vi "read full file.vi"(8 "error in":errorcluster, 11 "file path":path) -> (0 "error out":errorcluster, 2 "data":string)   [LabVIEW 2013, in "NISE Tools File IO.lvlib"]
doc: "Reads the full binary contents of a file."
uses:
  NISE Tools File IO.lvlib
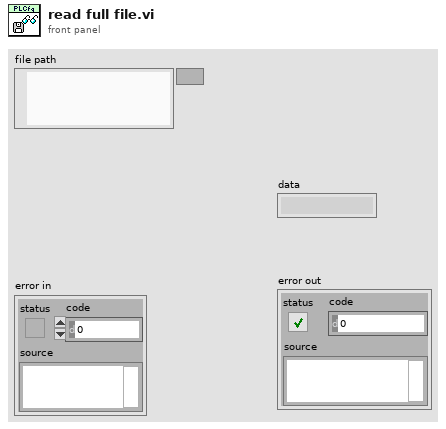
[diagram p1: front panel]
types:
  T1 = enum16{"open", "replace", "create", "open or create", "replace or create", "replace or create with confirmation"}
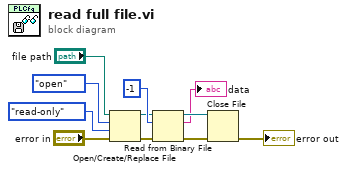
[diagram p0: block diagram]
diagram:
  n1 = Open/Create/Replace File(file path (use dialog)="file path", error in="error in", operation (0:open)=T1."open", access (0:read/write)=enum16{"read/write", "read-only", "write-only"}."read-only") -> (refnum out=w8:refnum<file>, error out=w6:errorcluster)  [unwired: 2 in, 1 out]
  n2 = Read from Binary File(8:w6, 10:-1 ("count"), 11:w8) -> (0:w5:errorcluster, 2:→"data":string, 3:w10:refnum<file>)  [unwired: 3 in, 1 out]
  n3 = Close File(refnum=w10, error in=w5) -> (error out=→"error out":errorcluster)  [unwired: 1 out]
